vi "Tacking Helper - Min_Max Angles.vi"(11 "Wind Direction (rad)":dbl) -> (1 "Irons/Tack\nIndicator":cluster{dbl, dbl, dbl, dbl}, 2 "Max Angle\nof Tack":dbl, 3 "Min Angle\nof Tack":dbl)   [LabVIEW 2011]
doc: "This vi takes the wind direction as an angle and returns the minimum and maximum tack vales as angles.\n\nThese are obtained by flipping the wind direction 180 degrees to find 'irons', then offsetting irons by 45 degrees on either side to get the angles at which to tack into the wind. The max value is always counter clockwise from irons and min is always clockwise, though sometimes max is less than min due to the jump from 360 to 0 degrees"
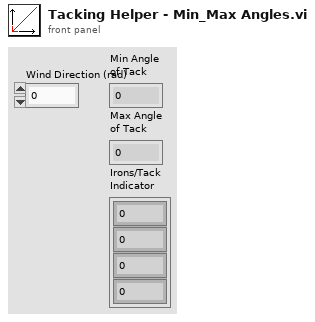
[diagram p1: front panel]
types:
  T1 = cluster{"Wind Direction (rad)":dbl, dbl, dbl, dbl}
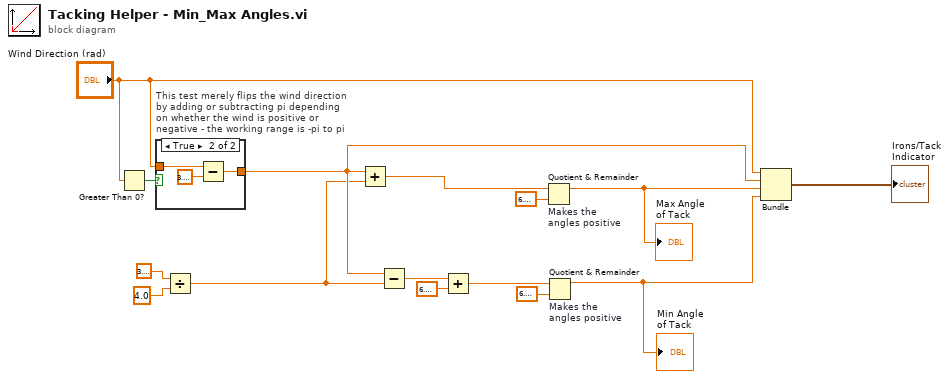
[diagram p0: block diagram]
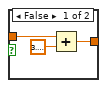
[diagram p2: hidden frame]
diagram:
  n1 = Greater Than 0?(x="Wind Direction (rad)") -> (x > 0?=w14:bool)
  n2 = case "This test merely flips the wind direction\nby adding or subtracting pi depending\non whether the wind is positive or\nnegative - the working range is -pi to pi" shown="True" w14 {
    tunnel: [w16 w20] -> w15
    tunnel: "Wind Direction (rad)" -> [w17 w19]
    frame False {
      n3 = Add(x=w17, y=3.141592653589793) -> (x+y=w16:dbl)
    }
    frame True {
      n4 = Subtract(x=w19, y=3.141592653589793) -> (x-y=w20:dbl)
    }
  }
  n5 = Divide(x=3.141592653589793, y=4.0) -> (x/y=w8:dbl)
  n6 = Add(x=w15, y=w8) -> (x+y=w7:dbl)
  n7 = Subtract(x=w15, y=w8) -> (x-y=w3:dbl)
  n8 = Add(x=w3, y=6.283185307179586) -> (x+y=w9:dbl)
  n9 = Quotient & Remainder "Makes the\nangles positive"(x=w7, y=6.283185307179586) -> (x-y*floor(x/y)=w11:dbl)  [unwired: 1 out]
  "Max Angle\nof Tack" <- w11
  n10 = Quotient & Remainder "Makes the\nangles positive"(x=w9, y=6.283185307179586) -> (x-y*floor(x/y)=w10:dbl)  [unwired: 1 out]
  "Min Angle\nof Tack" <- w10
  n11 = Bundle("Wind Direction (rad)"="Wind Direction (rad)", w15, w11, w10) -> (→"Irons/Tack\nIndicator":T1)  [unwired: 1 in]
